vi "CHAVEAMENTO.vi"() -> ()   [LabVIEW 2019]
uses:
  <vilib>/measure/NI_MABase.lvlib
panel:
  in  "Tab Control":enum32{"Page 1", "Page 2", "Page 3"}(tab)
  out "Waveform Chart 3":waveform(dbl)(graph)
  out "error out 3":errorcluster
  in  "error in (no error) 3":errorcluster
  out "Waveform Chart 2":waveform(dbl)(graph)
  out "Waveform Chart":waveform(dbl)(graph)
  in  "offset":dbl format="%0.2p"
  in  "sampling info":cluster{"Fs":dbl, "#s":dbl}={"Fs"=1000.0, "#s"=1000.0} {"Fs" format="%.2p"}
  in  "reset signal":bool
  in  "error in (no error)":errorcluster
  in  "phase":dbl format="%.2p"
  in  "amplitude":dbl=1.0 format="%0.2p"
  in  "frequency":dbl=10.0 format="%0.2p"
  out "error out":errorcluster
  out "error out 2":errorcluster
  in  "frequency 2":dbl=10.0 format="%0.2p"
  in  "amplitude 2":dbl=1.0 format="%0.2p"
  in  "phase 2":dbl format="%.2p"
  in  "error in (no error) 2":errorcluster
  in  "reset signal 2":bool
  in  "sampling info 2":cluster{"Fs":dbl, "#s":dbl}={"Fs"=1000.0, "#s"=1000.0} {"Fs" format="%.2p"}
  in  "offset 2":dbl format="%0.2p"
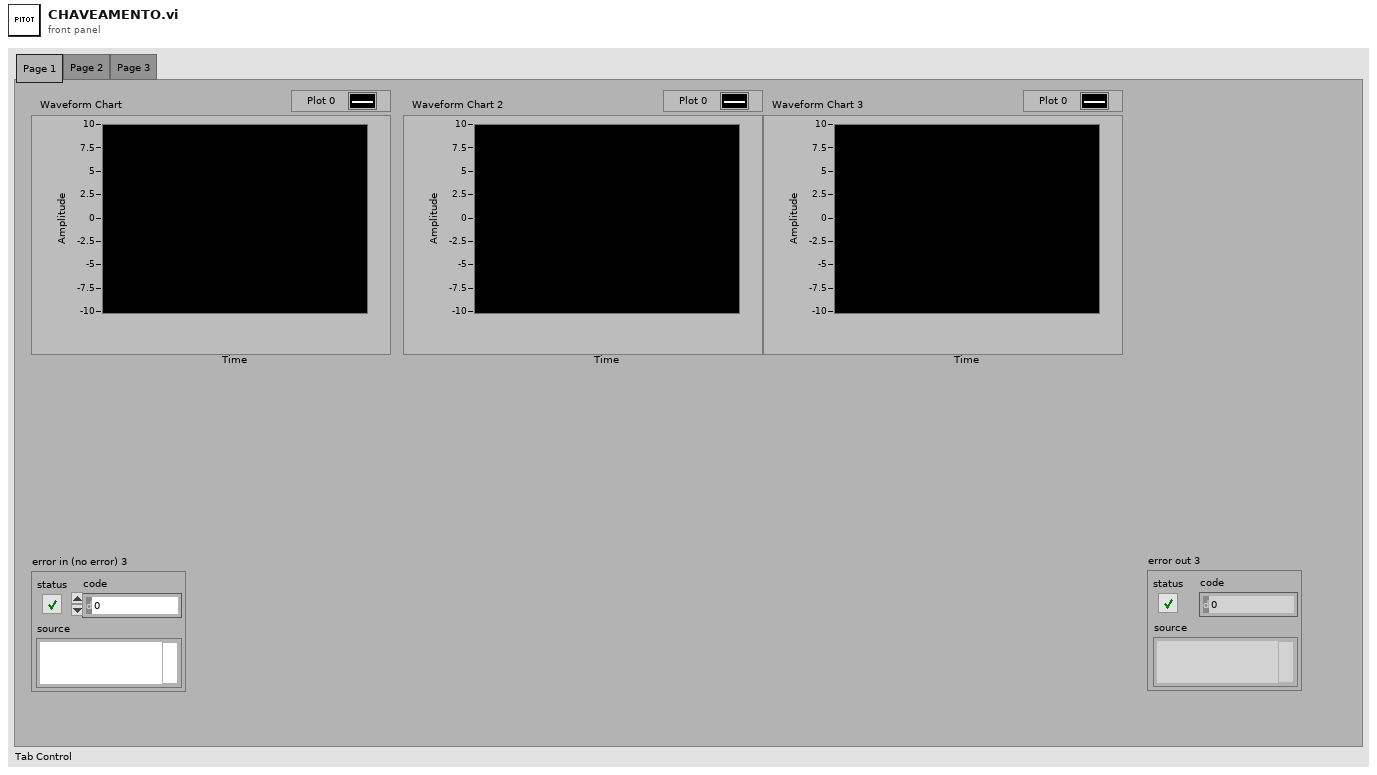
[diagram p1: front panel]
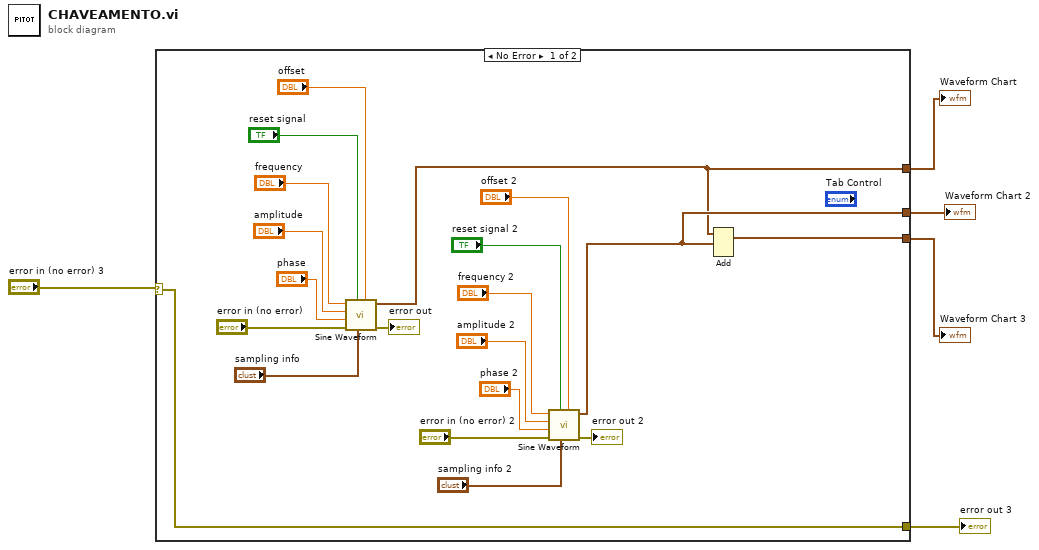
[diagram p0: block diagram]
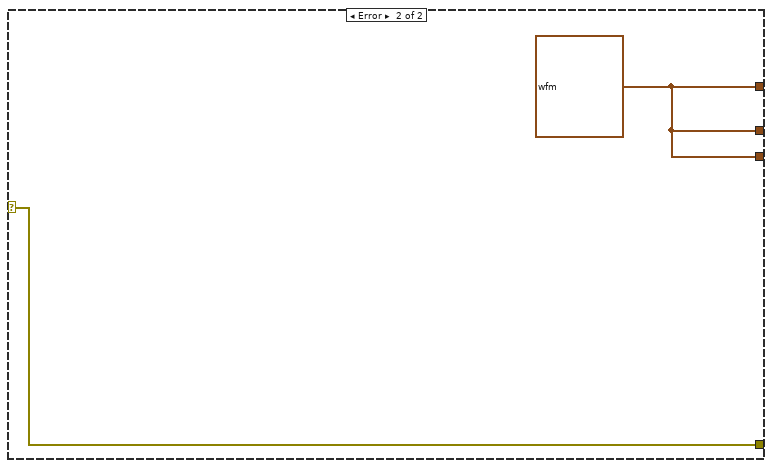
[diagram p2: hidden frame]
diagram:
  n1 = case shown="No Error" "error in (no error) 3" {
    selector: "error in (no error) 3" -> [w9 w27]
    tunnel: [w9 w27] -> w4
    tunnel: [w6 w26] -> w3
    tunnel: [w8 w26] -> w2
    tunnel: [w7 w26] -> w1
    frame No Error {
      n2 = call <vilib>:"Sine Waveform.vi"("offset"="offset", "sampling info"="sampling info", "reset signal"="reset signal", "error in (no error)"="error in (no error)", "phase"="phase", "amplitude"="amplitude", "frequency"="frequency") -> ("error out"=→"error out":errorcluster, "signal out"=w6:waveform(dbl))  [unwired: 3 in]
      n3 = call <vilib>:"Sine Waveform.vi"("offset"="offset 2", "sampling info"="sampling info 2", "reset signal"="reset signal 2", "error in (no error)"="error in (no error) 2", "phase"="phase 2", "amplitude"="amplitude 2", "frequency"="frequency 2") -> ("error out"=→"error out 2":errorcluster, "signal out"=w8:waveform(dbl))  [unwired: 3 in]
      n4 = Add(1:w8, 2:w6) -> (0:w7:waveform(dbl))  [unwired: 1 in, 1 out]
    }
    frame Error {
      w26 = waveform(dbl) {"t0"=timestamp(0 s since 1904-01-01), "dt"=1.0, "Y"=[]} ("signal out")
    }
  }
  "Waveform Chart" <- w3
  "Waveform Chart 2" <- w2
  "error out 3" <- w4
  "Waveform Chart 3" <- w1
